vi "main.vi"() -> ()   [LabVIEW 2022 SP3]
panel:
  out "Sampling frequency":dbl
  out "Scaled Waveform":dbl[](graph)
  in  "s/div":dbl format="%#_13g"
  in  "V/div":dbl=1.0
  in  "Control":T1(array[cluster])=[{"Device"=10, "Operation"=0, "Command/byte count"="OUTP:LOAD INF\nAPPL:SIN 1000,10,0"}, {"Device"=1, "Operation"=0, "Command/byte count"="HEAD OFF\nDAT:SOU CH1\nDAT:ENC ASCI\nDAT:WID 1\nDAT:STAR 1\nDAT:STOP 2500\nCH1:SCA 1\nHOR:MAI:SCA 250E-6\nCURV?"}, {"Device"=1, "Operation"=1, "Command/byte count"="15000"}] {"Operation" items=["write", "read"]; "Device" items=["DSO"=1, "AWG"=10]}
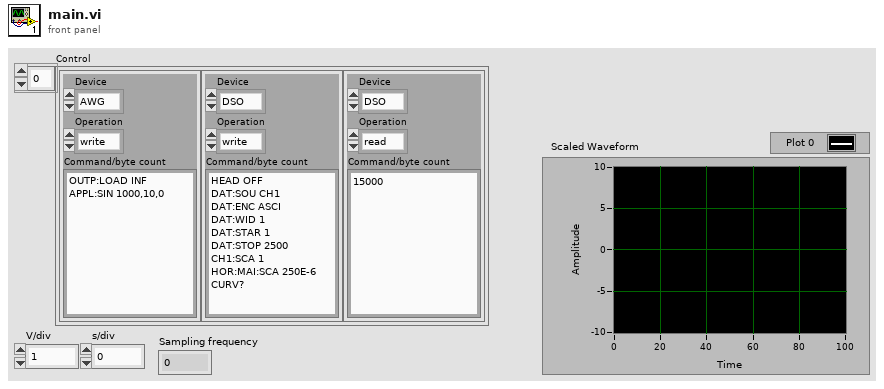
[diagram p1: front panel]
types:
  T1 = cluster{"Device":u16, "Operation":u16, "Command/byte count":string}[]
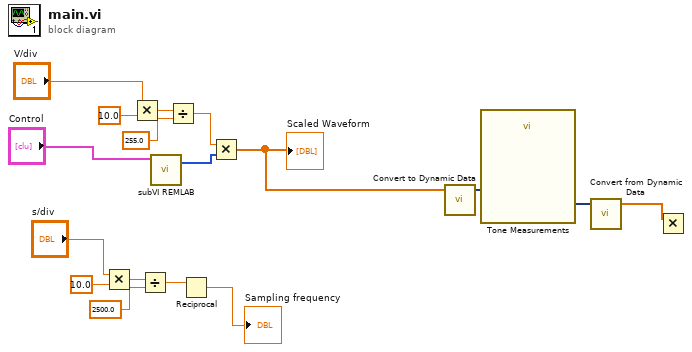
[diagram p0: block diagram]
diagram:
  n1 = Multiply(x="s/div", y=10.0) -> (x*y=w7:dbl)
  n2 = Multiply(x="V/div", y=10.0) -> (x*y=w15:dbl)
  n3 = Divide(x=w7, y=2500.0) -> (x/y=w4:dbl)
  n4 = call "subVI REMLAB.vi"("Control"="Control") -> ("Campioni Acquisiti"=w13:i32[])  [unwired: 3 in, 1 out]
  n5 = Divide(x=w15, y=255.0) -> (x/y=w12:dbl)
  n6 = Reciprocal(x=w4) -> (1/x=→"Sampling frequency":dbl)
  n7 = Multiply(x=w12, y=w13) -> (x*y=w10:dbl[])
  "Scaled Waveform" <- w10
  n8 = call "Convert to Dynamic Data"("Array"=w10) -> ("Dynamic Data Type"=w9:dynamicdata)  [unwired: 3 in]
  n9 = call "Tone Measurements"("Signals"=w9) -> ("Frequency"=w2:dynamicdata)  [unwired: 9 in, 1 out]
  n10 = call "Convert from Dynamic Data"("Dynamic Data Type"=w2) -> ("Array"=w1:dbl[])  [unwired: 3 in]
  n11 = Multiply(x=w1) -> ()  [unwired: 1 in, 1 out]
